vi "M06 Solar Cells v2.vi"(11 "EV3 in":T1) -> (3 "EV3 out":T1)   [LabVIEW 2016]
uses:
  <vilib>/NXT/Subs/LVHSConnector.ctl
  <vilib>/NXT/LegoClasses/BrickReference/BrickReference.lvclass
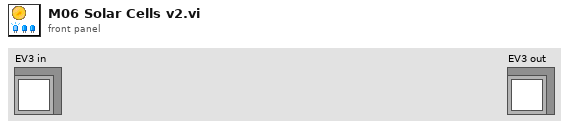
[diagram p1: front panel]
types:
  T1 = typedef "LVHSConnector.ctl" = refnum<class "BrickReference.lvclass">
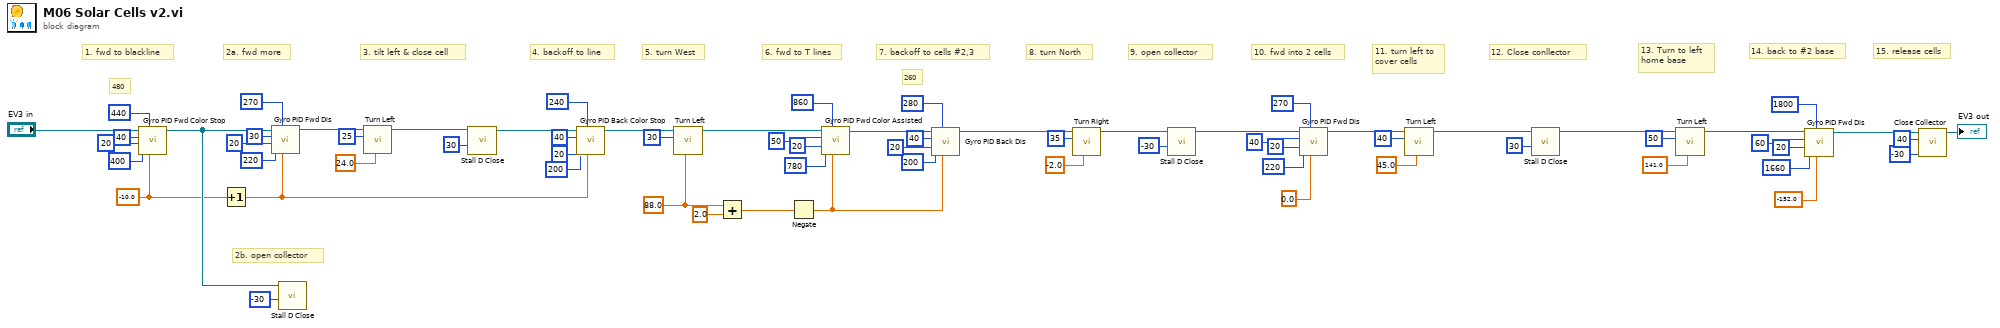
[diagram p0: block diagram]
diagram:
  w53 = sgl 88.0 ("Turning angle")
  w10 = sgl -10.0 ("Target angle")
  # "260"
  # "480"
  # "15. release cells"
  # "14. back to #2 base"
  # "13. Turn to left \nhome base"
  # "12. Close conllector"
  # "11. turn left to\ncover cells"
  # "10. fwd into 2 cells"
  # "9. open collector"
  # "8. turn North"
  # "7. backoff to cells #2,3"
  # "5. turn West"
  # "4. backoff to line"
  # "6. fwd to T lines"
  # "3. tilt left & close cell"
  # "2b. open collector"
  # "2a. fwd more"
  # "1. fwd to blackline"
  n1 = call "Gyro PID Fwd Color Stop.vi"("Target angle"=w10, "Threshold to Color"=440, "Threshold to slow"=400, "Min. speed"=20, "Max. speed"=40, "EV3 in"="EV3 in") -> ("EV3 out"=w30:T1)  [unwired: 5 in]
  n2 = Increment(x=w10) -> (x+1=w8:sgl)
  n3 = call "Gyro PID Fwd Dis.vi"("Target angle"=w8, "Threshold to stop"=270, "Threshold to slow"=220, "Min. speed"=20, "Max. speed"=30, "EV3 in"=w30) -> ("EV3 out"=w9:T1)  [unwired: 5 in]
  n4 = call "Stall D Close.vi"("Power"=i8 -30, "NXT/EV3"=w30) -> ()  [unwired: 9 in, 1 out]
  n5 = call "Turn Left.vi"("Turning angle"=sgl 24.0, "Motor B (right)"=i8 25, "EV3 in"=w9) -> ("EV3 out"=w7:T1)  [unwired: 8 in]
  n6 = call "Stall D Close.vi"("Power"=i8 30, "NXT/EV3"=w7) -> ("NXT/EV3"=w48:T1)  [unwired: 9 in]
  n7 = call "Gyro PID Back Color Stop.vi"("Target angle"=w8, "Threshold to Color"=240 ("Threshold to stop"), "Threshold to slow"=200, "Min. speed"=20, "Max. speed"=40, "EV3 in"=w48) -> ("EV3 out"=w29:T1)  [unwired: 5 in]
  n8 = call "Turn Left.vi"("Turning angle"=w53, "Motor B (right)"=i8 30, "EV3 in"=w29) -> ("EV3 out"=w45:T1)  [unwired: 8 in]
  n9 = Add(x=w53, y=sgl 2.0) -> (x+y=w55:sgl)
  n10 = Negate(x=w55) -> (-x=w23:sgl)
  n11 = call "Gyro PID Fwd Color Assisted.vi"("Target angle"=w23, "Threshold to Color"=860 ("Threshold to stop"), "Threshold to slow"=780, "Min. speed"=20, "Max. speed"=50, "EV3 in"=w45) -> ("EV3 out"=w42:T1)  [unwired: 5 in]
  n12 = call "Gyro PID Back Dis.vi"("Target angle"=w23, "Threshold to stop"=280, "Threshold to slow"=200, "Min. speed"=20, "Max. speed"=40, "EV3 in"=w42) -> ("EV3 out"=w28:T1)  [unwired: 5 in]
  n13 = call "Turn Right.vi"("Turning angle"=sgl -2.0, "Motor B (right)"=i8 35, "EV3 in"=w28) -> ("EV3 out"=w40:T1)  [unwired: 8 in]
  n14 = call "Stall D Close.vi"("Power"=i8 -30, "NXT/EV3"=w40) -> ("NXT/EV3"=w35:T1)  [unwired: 9 in]
  n15 = call "Gyro PID Fwd Dis.vi"("Target angle"=sgl 0.0, "Threshold to stop"=270, "Threshold to slow"=220, "Min. speed"=20, "Max. speed"=40, "EV3 in"=w35) -> ("EV3 out"=w33:T1)  [unwired: 5 in]
  n16 = call "Turn Left.vi"("Turning angle"=sgl 45.0, "Motor B (right)"=i8 40, "EV3 in"=w33) -> ("EV3 out"=w21:T1)  [unwired: 8 in]
  n17 = call "Stall D Close.vi"("Power"=i8 30, "NXT/EV3"=w21) -> ("NXT/EV3"=w18:T1)  [unwired: 9 in]
  n18 = call "Turn Left.vi"("Turning angle"=sgl 141.0, "Motor B (right)"=i8 50, "EV3 in"=w18) -> ("EV3 out"=w12:T1)  [unwired: 8 in]
  n19 = call "Gyro PID Fwd Dis.vi"("Target angle"=sgl -152.0, "Threshold to stop"=1800, "Threshold to slow"=1660, "Min. speed"=20, "Max. speed"=60, "EV3 in"=w12) -> ("EV3 out"=w4:T1)  [unwired: 5 in]
  n20 = call "Close Collector.vi"("Power"=i8 -30, "Rotation"=40, "EV3 in"=w4) -> ("EV3 out"=→"EV3 out":T1)  [unwired: 8 in]
